vi "DisposeCore.vi"(8 "error in (no error)":errorcluster, 11 "Creator in":refnum<class "Creator.lvclass">) -> (0 "error out":errorcluster, 3 "Creator out":refnum<class "Creator.lvclass">)   [LabVIEW 2020, in "FactoryMethod.lvlib" / "Creator.lvclass"]
uses:
  Creator.lvclass
  Private/TypeDef/privateDataDVR.ctl
  Private/TypeDef/privateData.ctl
  Product/Product.lvclass
  Creator.lvclass/Creator.ctl
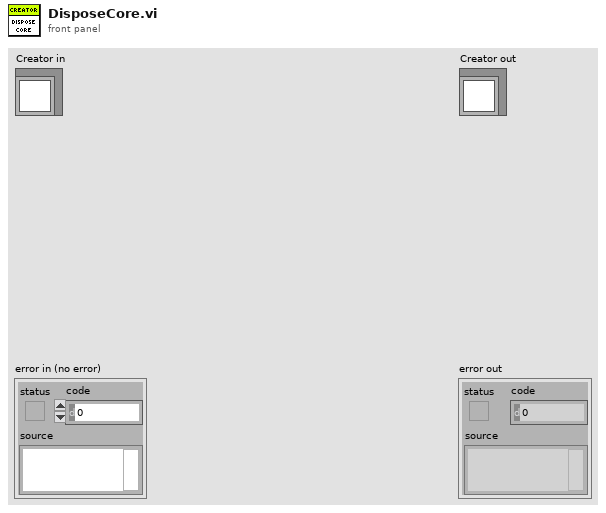
[diagram p1: front panel]
types:
  T1 = typedef "FactoryMethod.lvlib/Creator.lvclass/privateDataDVR.ctl" = refnum<data-value>
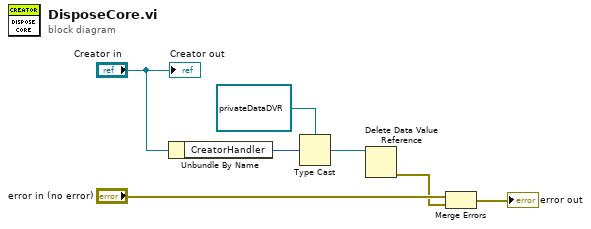
[diagram p0: block diagram]
diagram:
  n1 = Unbundle By Name("Creator in") -> ("CreatorHandler"=w6:u32)
  n2 = Type Cast(type=T1 refnum ("privateDataDVR"), x=w6) -> (*(type *) &x=w7:T1)
  n3 = Delete Data Value Reference(data value reference=w7) -> (error out=w1:errorcluster)  [unwired: 1 in, 1 out]
  n4 = Merge Errors("error in (no error)", w1) -> (→"error out":errorcluster)
  "Creator out" <- "Creator in"
